vi "Read shared variable refnum out.vi"(8 "error in (no error)":errorcluster, 11 "ibsen in":refnum<class "ibsen.lvclass">) -> (0 "error out":errorcluster, 2 "shared variable refnum out":refnum<k21>, 3 "ibsen out":refnum<class "ibsen.lvclass">)   [LabVIEW 2019, in "ibsen.lvlib" / "ibsen.lvclass"]
uses:
  ibsen.lvclass
  ibsen.lvclass/ibsen.ctl
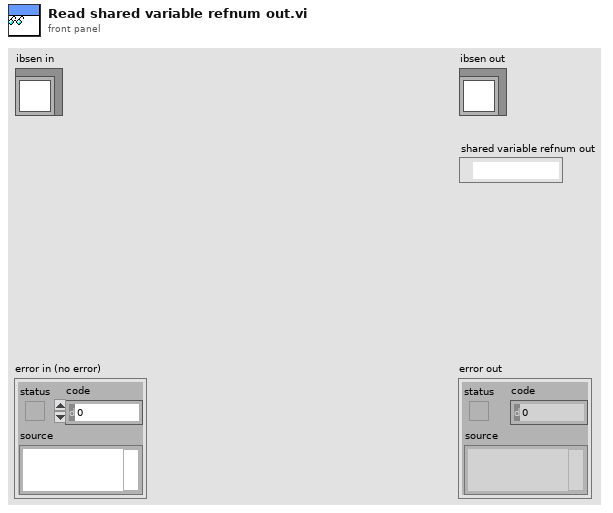
[diagram p1: front panel]
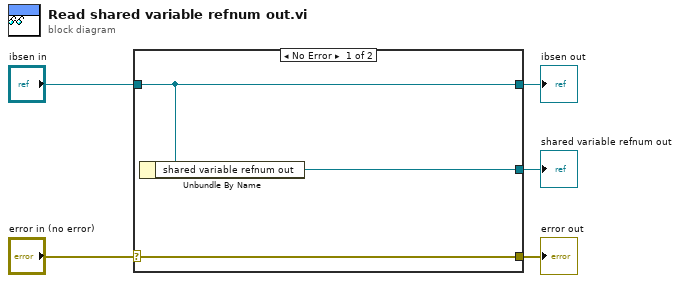
[diagram p0: block diagram]
diagram:
  n1 = case shown="No Error" "error in (no error)" {
    selector: "error in (no error)" -> [w8 w9]
    tunnel: [w8 w9] -> w4
    tunnel: [w7 w10] -> w2
    tunnel: "ibsen in" -> [w7 w10]
    tunnel: [w6 _] -> w1
    frame No Error {
      n2 = Unbundle By Name(w7) -> ("shared variable refnum out"=w6:refnum<k21>)
    }
    frame Error {
    }
  }
  "error out" <- w4
  "ibsen out" <- w2
  "shared variable refnum out" <- w1
